vi "updateSequence.vi"(8 "error in (no error)":errorcluster, 11 "Simon_Engine in":refnum<class "Simon_Engine.lvclass">) -> (0 "error out":errorcluster, 3 "Simon_Engine out":refnum<class "Simon_Engine.lvclass">)   [LabVIEW 2019, in "Simon_Engine.lvclass"]
doc: "Adds a new item to the sequence."
uses:
  Simon_Engine.lvclass
  LED/LED Class/LED.lvclass
  Simon_Engine.lvclass/Simon_Engine.ctl
  LED/LED Class/LED.lvclass/LED.ctl
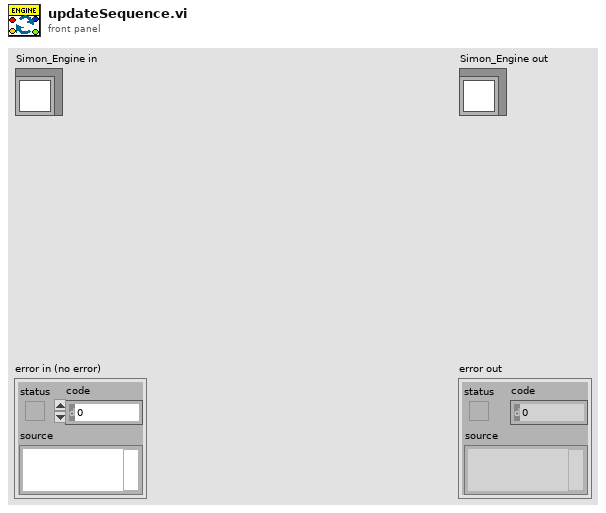
[diagram p1: front panel]
types:
  T1 = enum8{"Enabled", "Disabled", "Disabled and Grayed Out"}
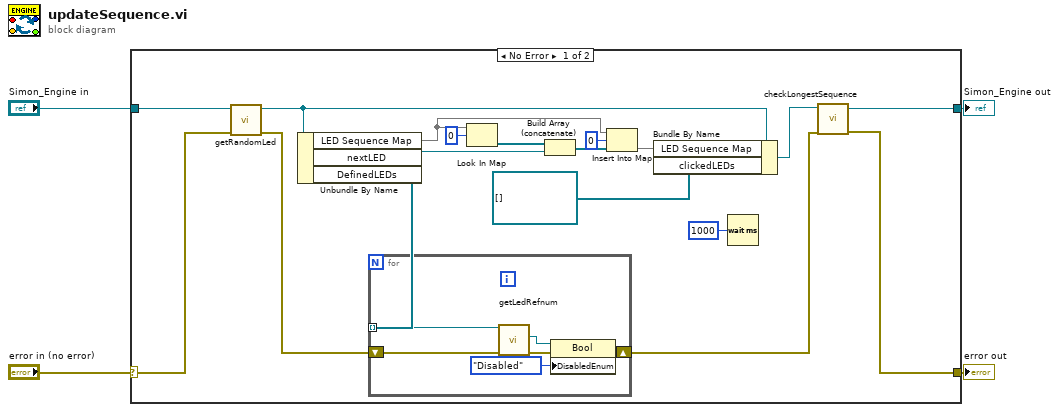
[diagram p0: block diagram]
diagram:
  n1 = case shown="No Error" "error in (no error)" {
    selector: "error in (no error)" -> [w22 w30]
    tunnel: [w15 w30] -> w3
    tunnel: [w13 w29] -> w1
    tunnel: "Simon_Engine in" -> [w20 w29]
    frame No Error {
      n2 = call "getRandomLed.vi"("error in (no error)"=w22, "Simon_Engine in"=w20) -> ("error out"=w21:errorcluster, "Simon_Engine out"=w19:refnum<class "Simon_Engine.lvclass">)  [unwired: 8 in]
      n3 = Unbundle By Name(w19) -> ("LED Sequence Map"=w7:map{u8, refnum<class "LED.lvclass">[]}, "nextLED"=w18:refnum<class "LED.lvclass">, "DefinedLEDs"=w11:refnum<class "LED.lvclass">[])
      n4 = for {
        shift-right: [w27] -> w12
        shift-left: w21 -> [w28]
        tunnel: w11 -> [w24] mode=indexing
        n5 = call "getLedRefnum.vi"("error in (no error)"=w28, "LED in"=w24) -> ("error out"=w26:errorcluster, "LED Refnum"=w25:refnum<vi>)  [unwired: 7 in, 1 out]
        n6 = property class="Bool"(reference=w25, error in=w26, "DisabledEnum"=T1."Disabled" ("Disabled")) -> (error out=w27:errorcluster)  [unwired: 1 out]
      }
      n7 = Look In Map(map=w7, key=u8 0) -> (value=w10:refnum<class "LED.lvclass">[])  [unwired: 1 in, 1 out]
      n8 = Build Array (concatenate)(w10, w18) -> (w6:refnum<class "LED.lvclass">[])
      n9 = Insert Into Map(map in=w7, key=u8 0, value=w6) -> (map out=w8:map{u8, refnum<class "LED.lvclass">[]})  [unwired: 2 out]
      n10 = Bundle By Name(cluster=w19, "LED Sequence Map"=w8, "clickedLEDs"=refnum<class "LED.lvclass">[] []) -> (w14:refnum<class "Simon_Engine.lvclass">)
      n11 = Wait (ms)(milliseconds to wait=u32 1000) -> ()  [unwired: 1 out]
      n12 = call-dynamic "checkLongestSequence.vi"("error in (no error)"=w12, "Simon_Engine in"=w14) -> ("error out"=w15:errorcluster, "Simon_Engine out"=w13:refnum<class "Simon_Engine.lvclass">)  [unwired: 8 in]
    }
    frame Error {
    }
  }
  "error out" <- w3
  "Simon_Engine out" <- w1
